vi "Scale Panel Bounds.vi"(7 "scale position? (F)":bool, 10 "scaling settings":T1={"scaling factor"={"horizontal"=1.0, "vertical"=1.0}, "scale text"=FALSE} {"scaling factor"."vertical" min=0.0; "scaling factor"."horizontal" min=0.0}, 11 "bounds in":T3) -> (3 "bounds out":T3)   [LabVIEW 2012, in "NI_SE_Front Panel Layout.lvlib"]
uses:
  NI_SE_Front Panel Layout.lvlib
  <vilib>/Utility/miscctls.llb/LVRectTypeDef.ctl
  Scaling Factor_Options.ctl
  XY Scaling Factor.ctl
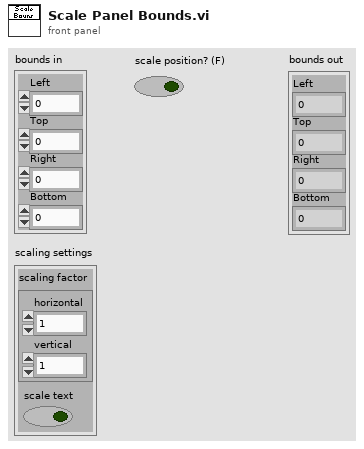
[diagram p1: front panel]
types:
  T1 = typedef "NI_SE_Front Panel Layout.lvlib/Scaling Factor_Options.ctl" = cluster{"scaling factor":T2, "scale text":bool}
  T2 = typedef "NI_SE_Front Panel Layout.lvlib/XY Scaling Factor.ctl" = cluster{"horizontal":dbl, "vertical":dbl}
  T3 = typedef "LVRectTypeDef.ctl" = cluster{"Left":i16, "Top":i16, "Right":i16, "Bottom":i16}
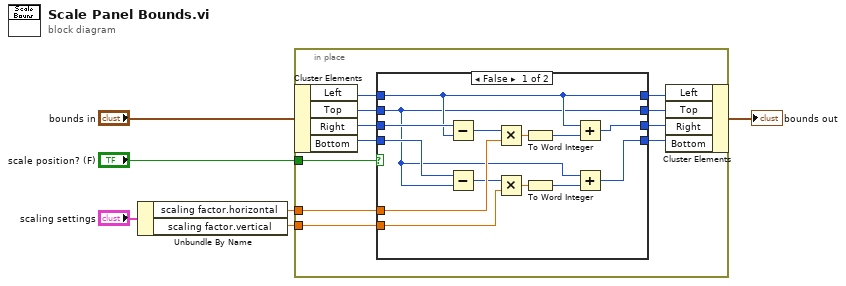
[diagram p0: block diagram]
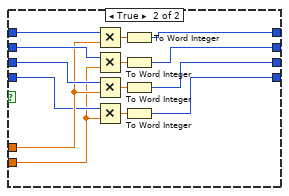
[diagram p2: hidden frame]
diagram:
  n1 = Unbundle By Name("scaling settings") -> ("scaling factor.horizontal"=w5:dbl, "scaling factor.vertical"=w4:dbl)
  n2 = in-place {
    in-place-border: w5 -> [w17]
    in-place-border: w4 -> [w16]
    in-place-border: "scale position? (F)" -> [w15]
    n3 = in-place-cluster #1("bounds in") -> ("Left"=w14:i16, "Top"=w13:i16, "Right"=w12:i16, "Bottom"=w11:i16)
    n4 = case shown="False" w15 {
      tunnel: w12 -> [w31 w38]
      tunnel: w17 -> [w29 w37]
      tunnel: w14 -> [w19 w44]
      tunnel: [w27 w32] -> w8
      tunnel: w11 -> [w25 w35]
      tunnel: w16 -> [w23 w34]
      tunnel: w13 -> [w18 w42]
      tunnel: [w20 w33] -> w7
      tunnel: [w19 w43] -> w10
      tunnel: [w18 w41] -> w9
      frame False {
        n5 = Subtract(x=w31, y=w19) -> (x-y=w30:i16)
        n6 = Subtract(x=w25, y=w18) -> (x-y=w24:i16)
        n7 = Multiply(x=w30, y=w29) -> (x*y=w28:dbl)
        n8 = Multiply(x=w24, y=w23) -> (x*y=w22:dbl)
        n9 = To Word Integer(number=w28) -> (16bit integer=w26:i16)
        n10 = To Word Integer(number=w22) -> (16bit integer=w21:i16)
        n11 = Add(x=w19, y=w26) -> (x+y=w27:i16)
        n12 = Add(x=w18, y=w21) -> (x+y=w20:i16)
      }
      frame True {
        n13 = Multiply(x=w44, y=w37) -> (x*y=w45:dbl)
        n14 = Multiply(x=w42, y=w34) -> (x*y=w39:dbl)
        n15 = Multiply(x=w38, y=w37) -> (x*y=w40:dbl)
        n16 = Multiply(x=w35, y=w34) -> (x*y=w36:dbl)
        n17 = To Word Integer(number=w45) -> (16bit integer=w43:i16)
        n18 = To Word Integer(number=w39) -> (16bit integer=w41:i16)
        n19 = To Word Integer(number=w40) -> (16bit integer=w32:i16)
        n20 = To Word Integer(number=w36) -> (16bit integer=w33:i16)
      }
    }
    n21 = in-place-cluster #1("Left"=w10, "Top"=w9, "Right"=w8, "Bottom"=w7) -> (→"bounds out":T3)
  }
